vi "Reset.vi"(8 "error in (no error)":errorcluster, 11 "handle in":u32) -> (0 "error out":errorcluster, 3 "handle out":u32)   [LabVIEW 2016, in "Photon Counter.lvlib" / "C8855-01.lvlib"]
doc: "Resets the settings for this unit.\n\n\n\nBOOL C8855API __stdcall C8855Reset( HANDLE hC8855 );"
uses:
  C8855-01.lvlib
  C8855-01api.dll
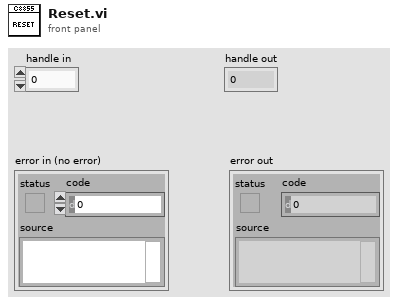
[diagram p1: front panel]
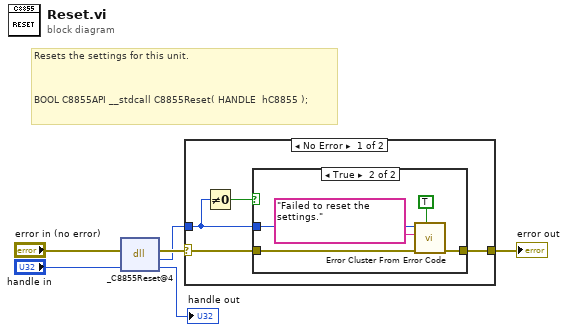
[diagram p0: block diagram]
diagram:
  # "Resets the settings for this unit.\n\n\n\nBOOL C8855API __stdcall C8855Reset( HANDLE  hC8855 );"
  n1 = dll-call lib="Z:/VM Shared Folder/Trace Grabber/Drivers/C8855-01/C8855-01api.dll" fn="_C8855Reset@4"(error in="error in (no error)", "Handle"="handle in") -> (error out=w4:errorcluster, "return type"=w3:i32, "Handle"=→"handle out":u32)  [unwired: 2 in, 1 out]
  n2 = case shown="No Error" w4 {
    selector: w4 -> [w9 w17]
    tunnel: w3 -> [w7 _]
    tunnel: [w8 w17] -> w2
    frame No Error {
      n3 = Not Equal To 0?(x=w7) -> (x != 0?=w10:bool)
      n4 = case shown="True" w10 {
        tunnel: w9 -> [w11 w15]
        tunnel: [w11 w14] -> w8
        tunnel: w7 -> [_ w13]
        frame False {
        }
        frame True {
          n5 = call <vilib>:"Error Cluster From Error Code.vi"("show call chain? (False)"=TRUE, "error in (no error)"=w15, "error message (\"\")"="Failed to reset the settings." ("error message (\"\")"), "error code (0)"=w13) -> ("error out"=w14:errorcluster)  [unwired: 5 in]
        }
      }
    }
    frame Error {
    }
  }
  "error out" <- w2
